vi "fbg_force_control_ui.vi"(1 "Goal Position IN":dbl[][](array[numeric])) -> (8 "Goal Position OUT":dbl[][](array[numeric]))   [LabVIEW 2013]
uses:
  <vilib>/Analysis/Matrix/NI_Matrix.lvlib
  force_control_globals.vi
  <vilib>/Analysis/NI_AALBase.lvlib
  <vilib>/Analysis/Matrix/Numeric/Conversions/Array To Matrix - RA2.vi
  <vilib>/Analysis/baseanly.llb/Vector x A.vi
panel:
  out "Force IN":dbl[](array[numeric])
  in  "Rotate FBG Output":bool=TRUE caption="FBG Enabled"
  in  "FBG Input":dbl[](array[numeric])=[0.0, 0.0, 0.0]
  in  "Override FBG":bool caption="FBG Enabled"
  in  "FBG Scaling":dbl=1.0
  out "FBG Enabled":bool=TRUE
  out "Load Cell Enabled":bool=TRUE
  out "Force Control Active":bool
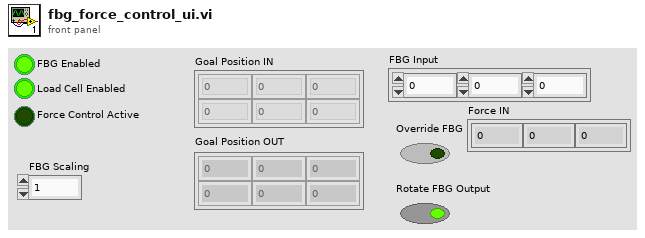
[diagram p1: front panel]
types:
  T1 = typedef "NI_Matrix.lvlib/RealMatrix.ctl" = dbl[][]
  T2 = enum16{"Setpoint", "One Way Threshold", "Two Way Threshold"}
  T3 = enum16{"Translation", "Tip Position", "Rotation"}
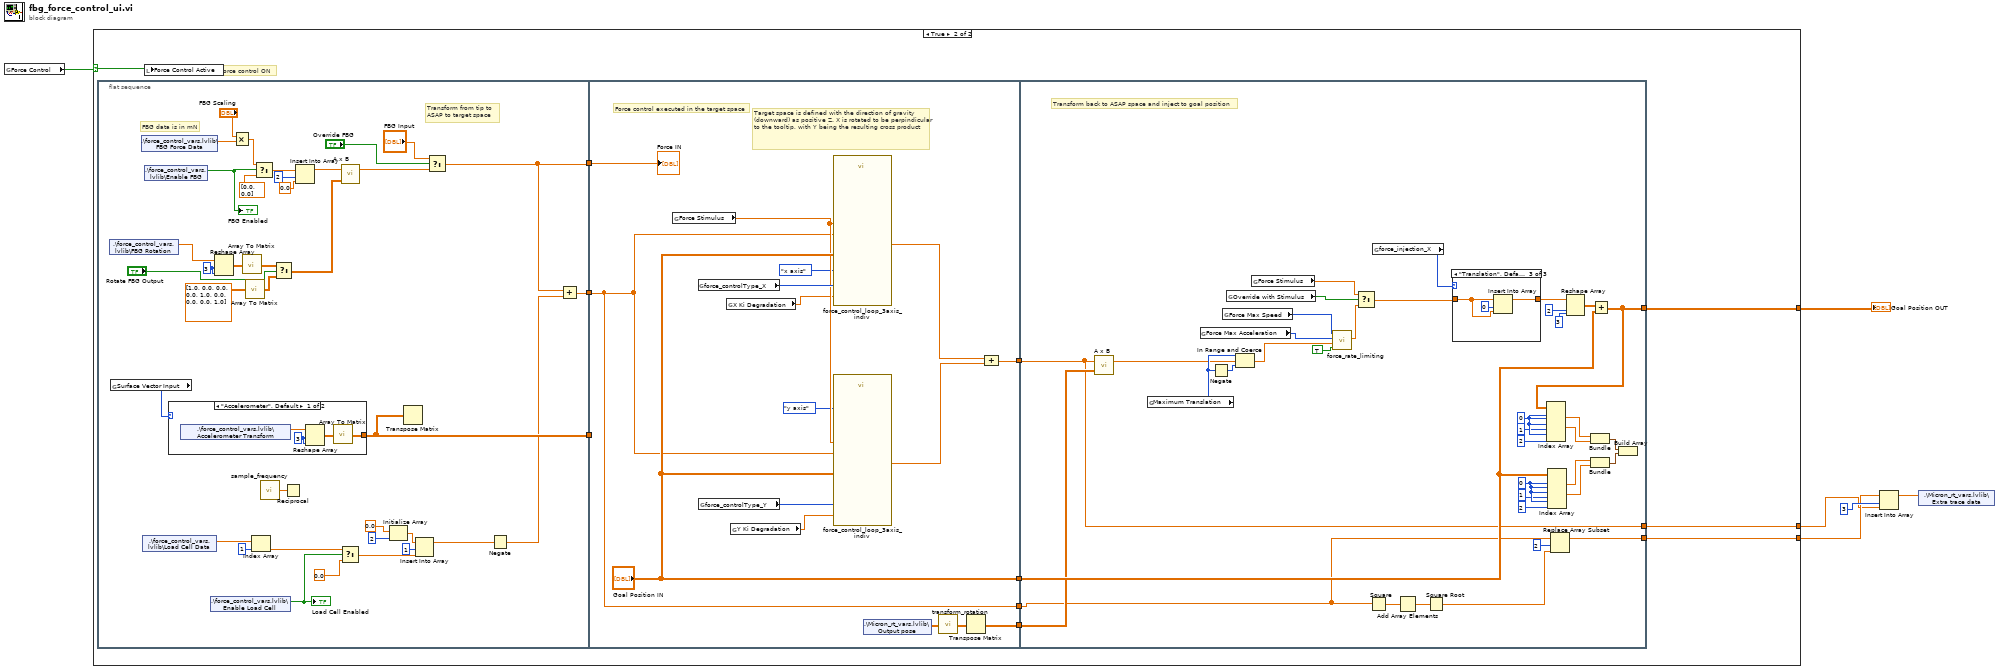
[diagram p0: block diagram]
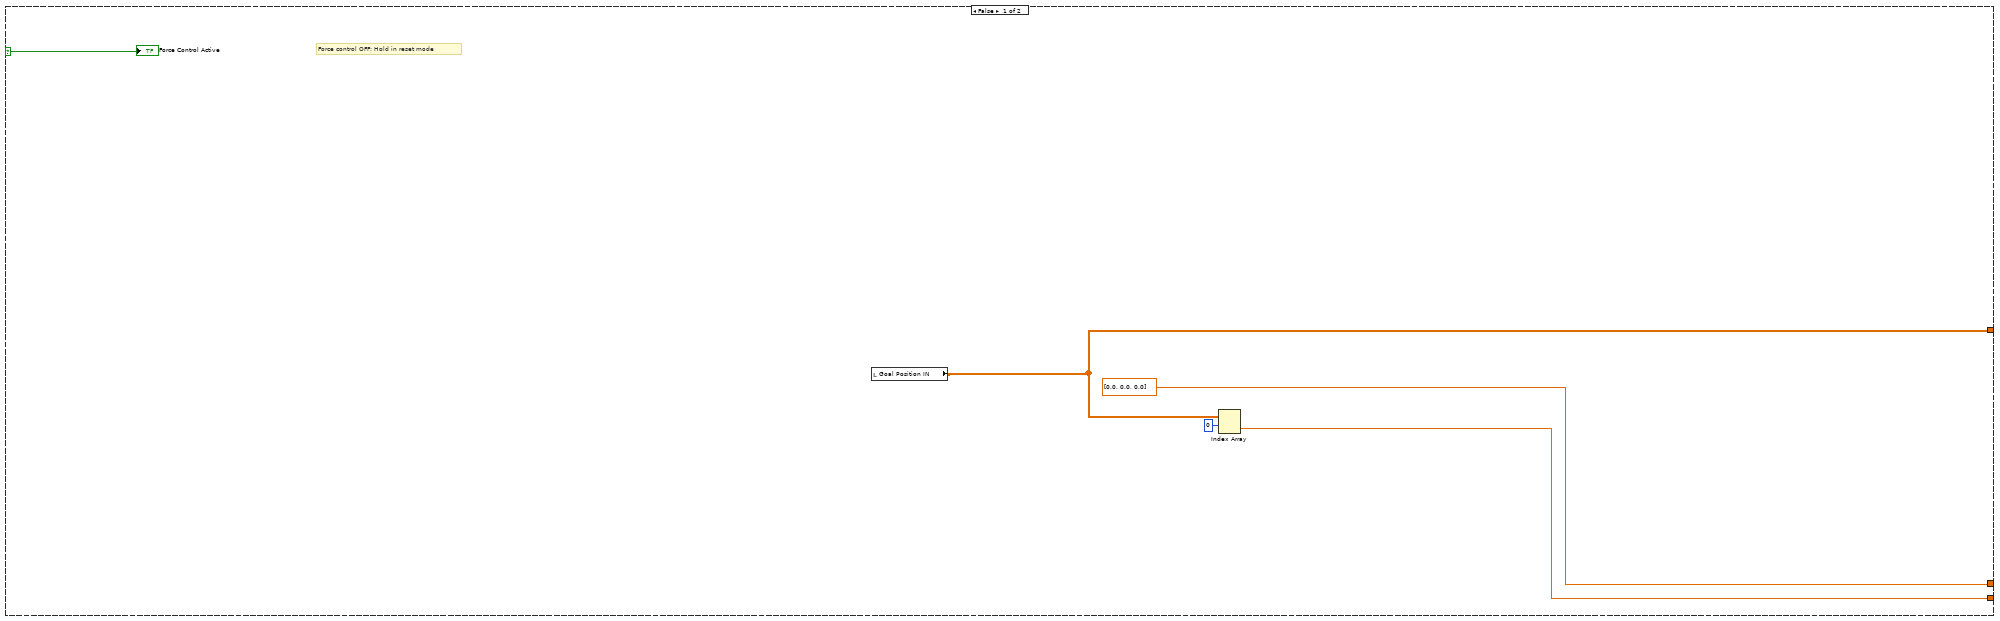
[diagram p2: hidden frame]
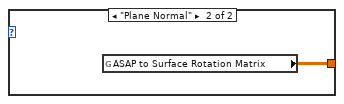
[diagram p3: hidden frame]
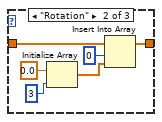
[diagram p5: hidden frame]
diagram:
  n1 = global read "force_control_globals.vi" "Force Control"() -> (w5:bool)
  n2 = case shown="True" w5 {
    selector: w5 -> [w11 w22]
    tunnel: [w7 w21] -> w6
    tunnel: [w9 w15] -> w2
    tunnel: [dbl[] [0.0, 0.0, 0.0] w19] -> w1
    frame False {
      # "Force control OFF: Hold in reset mode"
      n3 = local read "Goal Position IN"() -> (w7:dbl[][])
      n4 = Index Array(array=w7, index (row)=0) -> (element=w9:dbl[])  [unwired: 1 in]
      "Force Control Active" <- w11
    }
    frame True {
      # "Force control ON"
      n5 = flat-sequence {
        tunnel: [w26] -> w20
        tunnel: [w30] -> w17
        tunnel: [w25] -> w12
        tunnel: w20 -> [w65]
        tunnel: [w79] -> w18
        tunnel: w17 -> [_]
        tunnel: [w65] -> w16
        tunnel: ["Goal Position IN"] -> w14
        tunnel: [w69] -> w13
        tunnel: w12 -> [w72]
        tunnel: [w102] -> w21
        tunnel: [w81] -> w15
        tunnel: [w88] -> w19
        tunnel: w18 -> [w88]
        tunnel: w16 -> [w82]
        tunnel: w14 -> [w97]
        tunnel: w13 -> [w89]
        frame #0 {
          w38 = 3 ("dimension size")
          # "FBG data is in mN"
          # "Transform from tip to \nASAP to target space"
          n6 = shared-variable ".\\force_control_vars.lvlib\\FBG Rotation"() -> (w37:dbl[])  [unwired: 1 in, 1 out]
          n7 = global read "force_control_globals.vi" "Surface Vector Input"() -> (w51:enum16{"Accelerometer", "Plane Normal"})
          n8 = shared-variable ".\\force_control_vars.lvlib\\FBG Force Data"() -> (w40:dbl[])  [unwired: 1 in, 1 out]
          n9 = shared-variable ".\\force_control_vars.lvlib\\Load Cell Data"() -> (w53:dbl[])  [unwired: 1 in, 1 out]
          n10 = shared-variable ".\\force_control_vars.lvlib\\Enable FBG"() -> (w59:bool)  [unwired: 1 in, 1 out]
          "FBG Enabled" <- w59
          n11 = case shown="\"Accelerometer\", Default" w51 {
            tunnel: [w61 w64] -> w30
            frame "Accelerometer", Default {
              w60 = 3 ("dimension size")
              n12 = shared-variable ".\\force_control_vars.lvlib\\Accelerometer Transform"() -> (w63:dbl[])  [unwired: 1 in, 1 out]
              n13 = Reshape Array(w63, w60, w60) -> (w62:dbl[][])
              n14 = call-poly <vilib>:"Array To Matrix.vi"("Real 2D Array"=w62) -> ("Real Matrix"=w61:T1)
            }
            frame "Plane Normal" {
              n15 = global read "force_control_globals.vi" "ASAP to Surface Rotation Matrix"() -> (w64:T1)
            }
          }
          n16 = shared-variable ".\\force_control_vars.lvlib\\Enable Load Cell"() -> (w54:bool)  [unwired: 1 in, 1 out]
          "Load Cell Enabled" <- w54
          n17 = Reshape Array(w37, w38, w38) -> (w39:dbl[][])
          n18 = Multiply ("Multiply.vi")(x="FBG Scaling", y=w40) -> (x*y=w31:dbl[])
          n19 = call-poly <vilib>:"Array To Matrix.vi"("Real 2D Array"=w39) -> ("Real Matrix"=w36:T1)
          n20 = call-poly <vilib>:"Array To Matrix.vi"("Real 2D Array"=dbl[][] [[1.0, 0.0, 0.0], [0.0, 1.0, 0.0], [0.0, 0.0, 1.0]]) -> ("Real Matrix"=w34:T1)
          n21 = Index Array(array=w53, index=1) -> (element=w45:dbl)
          n22 = Select(t=w31, s=w59, f=sgl[] [0.0, 0.0]) -> (s? t:f=w50:dbl[])
          n23 = call "sample_frequency.vi"() -> ("Sample frequency"=w44:dbl)
          n24 = Select(t=w36, s="Rotate FBG Output", f=w34) -> (s? t:f=w35:T1)
          n25 = Reciprocal(x=w44) -> ()  [unwired: 1 out]
          n26 = Insert Into Array(array=w50, index=2, new element=sgl 0.0 ("new element/subarray")) -> (w29:dbl[])
          n27 = call-poly <vilib>:"A x B.vi"("Matrix A"=w35, "Vector V'"=w29) -> ("V' x A"=w28:dbl[])  [unwired: 1 out]
          n28 = Select(t=w45, s=w54, f=0.0 ("lower limit")) -> (s? t:f=w55:dbl)
          n29 = Initialize Array(sgl 0.0, 2) -> (w57:sgl[])
          n30 = Transpose Matrix(1:w30) -> ()  [unwired: 1 out]
          n31 = Insert Into Array(array=w57, index=1, new element=w55) -> (w24:sgl[])
          n32 = Select(t="FBG Input", s="Override FBG", f=w28) -> (s? t:f=w25:dbl[])
          n33 = Negate(x=w24) -> (-x=w23:sgl[])
          n34 = Add(x=w25, y=w23) -> (x+y=w26:dbl[])
        }
        frame #1 {
          # "Target space is defined with the direction of gravity (downward) as positive Z. X is rotated to be perpindicular to the tooltip, with Y being the resulting cross product"
          # "Force control executed in the target space"
          n35 = global read "force_control_globals.vi" "Force Stimulus"() -> (w75:dbl[])
          n36 = global read "force_control_globals.vi" "force_controlType_X"() -> (w80:T2)
          n37 = global read "force_control_globals.vi" "force_controlType_Y"() -> (w76:T2)
          n38 = global read "force_control_globals.vi" "X Ki Degradation"() -> (w67:dbl)
          n39 = global read "force_control_globals.vi" "Y Ki Degradation"() -> (w68:dbl)
          n40 = call "force_control_loop_3axis_indiv.vi"("Force In"=w65, "Goal Position IN"="Goal Position IN", "Force Stimulus"=w75, "Control Axis"=enum16{"x axis", "y axis", "z axis"}."x axis", "Force Control Type"=w80, "Ki Degradation"=w67) -> ("Force Position Out"=w78:dbl[])  [unwired: 8 in, 1 out]
          n41 = call "force_control_loop_3axis_indiv.vi"("Force In"=w65, "Goal Position IN"="Goal Position IN", "Force Stimulus"=w75, "Control Axis"=enum16{"x axis", "y axis", "z axis"}."y axis", "Force Control Type"=w76, "Ki Degradation"=w68) -> ("Force Position Out"=w66:dbl[])  [unwired: 8 in, 1 out]
          n42 = shared-variable ".\\Micron_rt_vars.lvlib\\Output pose"() -> (w71:sgl[][])  [unwired: 1 in, 1 out]
          n43 = call "transform_rotation.vi"("Transform"=w71) -> ("Rotation"=w70:T1)  [unwired: 4 in]
          n44 = Transpose Matrix(1:w70) -> (0:w69:T1)
          n45 = Compound Arithmetic op=ADD(w78, w66) -> (w79:dbl[])
          "Force IN" <- w72
        }
        frame #2 {
          w109 = 0 ("index")
          w113 = 0 ("index")
          # "Transform back to ASAP space and inject to goal position"
          n46 = call-poly <vilib>:"A x B.vi"("Matrix A"=w89, "Vector V'"=w88) -> ("V' x A"=w87:dbl[])  [unwired: 1 out]
          n47 = global read "force_control_globals.vi" "Maximum Translation"() -> (w93:i32)
          n48 = global read "force_control_globals.vi" "Force Max Acceleration"() -> (w95:i32)
          n49 = Negate(x=w93) -> (-x=w101:i32)
          n50 = global read "force_control_globals.vi" "Force Max Speed"() -> (w96:i32)
          n51 = global read "force_control_globals.vi" "Override with Stimulus"() -> (w94:bool)
          n52 = In Range and Coerce(upper limit=w93, x=w87, lower limit=w101) -> (coerced(x)=w100:dbl[])  [unwired: 1 out]
          n53 = global read "force_control_globals.vi" "Force Stimulus"() -> (w90:dbl[])
          n54 = call "force_rate_limiting.vi"("Rate Limiting"=TRUE, "Link goal"=w100, "force max accel"=w95, "force max vel"=w96) -> ("Substituted goal"=w98:sgl[])  [unwired: 7 in]
          n55 = Select(t=w90, s=w94, f=w98) -> (s? t:f=w91:dbl[])
          n56 = Square(x=w82) -> (x^2=w85:dbl[])
          n57 = global read "force_control_globals.vi" "force_injection_X"() -> (w92:T3)
          n58 = Add Array Elements(numeric array=w85) -> (sum=w86:dbl)
          n59 = Square Root(x=w86) -> (sqrt(x)=w83:dbl)
          n60 = case shown="\"Translation\", Default" w92 {
            tunnel: [w119 w124 w127] -> w116
            tunnel: w91 -> [w119 w123 w126]
            frame "Tip Position" {
            }
            frame "Rotation" {
              n61 = Initialize Array(0.0 ("element"), 3 ("dimension size")) -> (w122:dbl[])
              n62 = Insert Into Array(array=w123, index=0, new element=w122) -> (w124:dbl[])
            }
            frame "Translation", Default {
              n63 = Insert Into Array(array=w126, index=0, new element=w126) -> (w127:dbl[])
            }
          }
          n64 = Index Array(array=w97, index (row) #1=w109, index (col) #1=w109, index (row) #2=w109, index (col) #2=1 ("length"), index (row) #3=w109, index (col) #3=2 ("length")) -> (element #1=w105:dbl, element #2=w104:dbl)  [unwired: 1 out]
          n65 = Replace Array Subset(array=w82, new element=w83, index=2) -> (w81:dbl[])
          n66 = Reshape Array(w116, 2, 3) -> (w103:dbl[][])
          n67 = Bundle("Numeric"=w105, "Numeric"=w104) -> (w115:cluster{"Numeric":dbl, "Numeric":dbl})  [unwired: 1 in]
          n68 = Add ("Add.vi")(x=w103, y=w97) -> (x+y=w102:dbl[][])
          n69 = Index Array(array=w102, index (row) #1=w113, index (col) #1=w113, index (row) #2=w113, index (col) #2=1 ("length"), index (row) #3=w113, index (col) #3=2 ("length")) -> (element #1=w107:dbl, element #2=w106:dbl)  [unwired: 1 out]
          n70 = Bundle(w107, w106) -> (w114:cluster{dbl, dbl})  [unwired: 1 in]
          n71 = Build Array(w114, w115) -> ()  [unwired: 1 out]
        }
      }
      n72 = local write "Force Control Active"(w22) -> ()
    }
  }
  "Goal Position OUT" <- w6
  n73 = Insert Into Array(array=w2, index=3, new element=w1) -> (w3:dbl[])
  n74 = shared-variable ".\\Micron_rt_vars.lvlib\\Extra trace data"(w3) -> ()  [unwired: 1 in, 1 out]
